vi "ConnectOnly.vi"(8 "error in (no error)":errorcluster) -> (0 "error out":errorcluster, 3 "Success":bool)   [LabVIEW 2015, in "Tool Interface.lvlib"]
uses:
  Tool Interface.lvlib
  GLOB - Configuration Options.vi
  <resource>/objmgr/ni.dex.rc
panel:
  out "Writer Connected":bool
  out "Writer Endpoint Name":string
  out "Reader Connected":bool
  out "Reader Endpoint Name":string
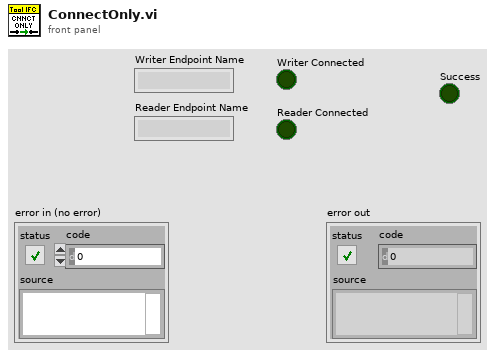
[diagram p1: front panel]
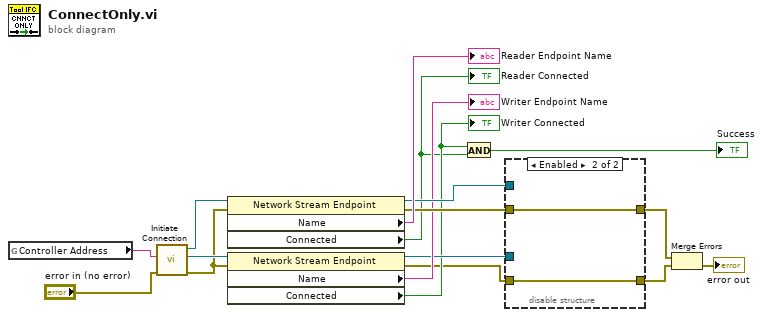
[diagram p0: block diagram]
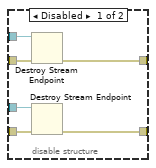
[diagram p2: hidden frame]
diagram:
  n1 = global read "GLOB - Configuration Options.vi" "Controller Address"() -> (w17:string)
  n2 = call "Initiate Connection.vi"("error in (no error)"="error in (no error)", "Controller Address"=w17) -> ("error out"=w12:errorcluster, "writer endpoint"=w13:refnum<k21>, "reader endpoint"=w14:refnum<k21>)  [unwired: 7 in]
  n3 = property class="Network Stream Endpoint"(reference=w14, error in=w12) -> (reference out=w11:refnum<k21>, error out=w10:errorcluster, "Name"=→"Reader Endpoint Name":string, "Connected"=w3:bool)
  "Reader Connected" <- w3
  n4 = property class="Network Stream Endpoint"(reference=w13, error in=w12) -> (reference out=w5:refnum<k21>, error out=w1:errorcluster, "Name"=→"Writer Endpoint Name":string, "Connected"=w4:bool)
  "Writer Connected" <- w4
  n5 = And(x=w4, y=w3) -> (x .and. y?=→"Success":bool)
  n6 = disable-structure shown="Enabled" {
    disable-tunnel: w11 -> [w23 _]
    disable-tunnel: w5 -> [w22 _]
    disable-tunnel: w10 -> [w21 w25]
    disable-tunnel: w1 -> [w20 w24]
    disable-tunnel: [w19 w24] -> w8
    disable-tunnel: [w18 w25] -> w7
    frame Disabled {
      n7 = Destroy Stream Endpoint(8:w21, 11:w23) -> (0:w18:errorcluster)
      n8 = Destroy Stream Endpoint(8:w20, 11:w22) -> (0:w19:errorcluster)
    }
    frame Enabled {
    }
  }
  n9 = Merge Errors(w7, w8) -> (→"error out":errorcluster)
